vi "OSP_from_cmd.vi"() -> ()   [LabVIEW 2019]
panel:
  out "Return code":i32
  in  "Path Control 2":path
  out "Image":T1(plugin-control)
  in  "Path Control":path
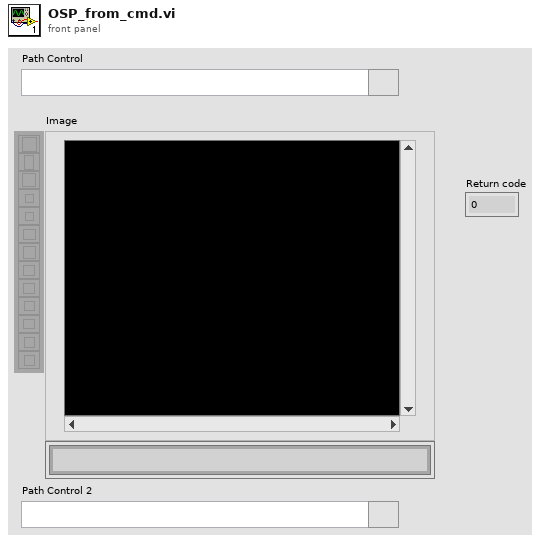
[diagram p1: front panel]
types:
  T1 = typedef "IMAQ Image.ctl" = refnum<image>
  T2 = typedef "Image Type" = u32
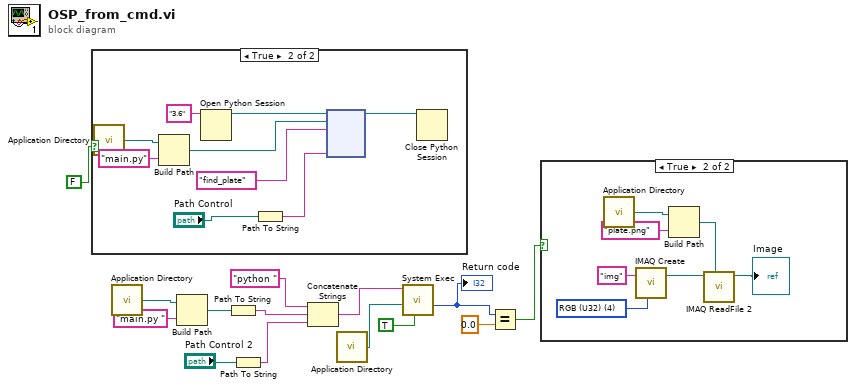
[diagram p0: block diagram]
diagram:
  n1 = case shown="True" FALSE {
    frame False {
    }
    frame True {
      n2 = call <vilib>:"Application Directory.vi"() -> ("Application Directory"=w18:path)
      n3 = Build Path(base path=w18, name or relative path="main.py") -> (appended path=w16:path)
      n4 = Open Python Session(python version="3.6" ("Python version")) -> (session out=w22:refnum<k35>)  [unwired: 2 in, 1 out]
      n5 = Path To String(path="Path Control") -> (string=w19:string)
      n6 = node(w22, w16, "find_plate" ("function name"), w19) -> (w21:refnum<k35>)  [unwired: 4 in, 3 out]
      n7 = Close Python Session(session in=w21) -> ()  [unwired: 1 in, 1 out]
    }
  }
  n8 = call <vilib>:"Application Directory.vi"() -> ("Application Directory"=w14:path)
  n9 = Build Path(base path=w14, name or relative path="main.py ") -> (appended path=w12:path)
  n10 = Path To String(path=w12) -> (string=w10:string)
  n11 = Path To String(path="Path Control 2") -> (string=w8:string)
  n12 = Concatenate Strings("python " ("string"), w10, w8) -> (w3:string)
  n13 = call <vilib>:"Application Directory.vi"() -> ("Application Directory"=w7:path)
  n14 = call <vilib>:"System Exec.vi"("run minimized? (F)"=TRUE, "working directory"=w7, "command line"=w3) -> ("return code"=w2:i32)  [unwired: 5 in, 3 out]
  "Return code" <- w2
  n15 = Equal?(x=w2, y=0.0) -> (x = y?=w4:bool)
  n16 = case shown="True" w4 {
    frame False {
    }
    frame True {
      w29 = T2 4 items=["Grayscale (U8)", "Grayscale (I16)", "Grayscale (SGL)", "Complex (CSG)", "RGB (U32)", "HSL (U32)", "RGB (U64)", "Grayscale (U16)"] ("Image Type")
      n17 = call <vilib>:"Application Directory.vi"() -> ("Application Directory"=w26:path)
      n18 = call "IMAQ Create"("Image Name"="img", "Image Type"=w29) -> ("New Image"=w28:T1)  [unwired: 3 in, 1 out]
      n19 = Build Path(base path=w26, name or relative path="plate.png") -> (appended path=w24:path)
      n20 = call "IMAQ ReadFile 2"("File Path"=w24, "Image"=w28) -> ("Image Out"=→"Image":T1)  [unwired: 5 in, 4 out]
    }
  }
